vi "Drive Modifications.vi"(1 "Drive Info In":T1) -> (0 "Drive Info Out":T1)   [LabVIEW 2013]
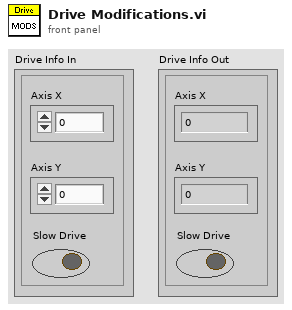
[diagram p1: front panel]
types:
  T1 = cluster{"Axis X":dbl, "Axis Y":dbl, "Slow Drive":bool}
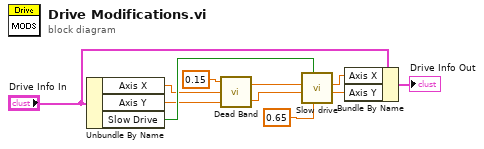
[diagram p0: block diagram]
diagram:
  n1 = Unbundle By Name("Drive Info In") -> ("Axis X"=w2:dbl, "Axis Y"=w1:dbl, "Slow Drive"=w11:bool)
  n2 = call "Dead Band.vi"("Axis 2 In"=w1, "Axis 1 In"=w2, "Dead Band"=0.15) -> ("Axis 2 Out"=w4:dbl, "Axis 1 Out"=w5:dbl)
  n3 = call "Slow drive.vi"("Slow drive to"=0.65, "Slow?"=w11, "Y-Axis"=w4, "X-Axis"=w5) -> ("Y - Axis out"=w6:dbl, "X-Axis out"=w7:dbl)  [unwired: 6 in]
  n4 = Bundle By Name(cluster="Drive Info In", "Axis X"=w7, "Axis Y"=w6) -> (→"Drive Info Out":T1)
